vi "PicoErrorHandler2.vi"(7 "Mode":u16(ring) items=["Dialog On Error", "no dialog - CloseUnit and Stop", "no dialog - Continue", "no dialog - Stop"], 8 "error in (no error)":errorcluster={"status"=FALSE, "code"=0, "source"="0"}, 9 "PICO_STATUS in":T1={"status"=FALSE, "code"=0, "source"="NC"}, 10 "Default handle":i16=16384, 11 "handle In":i16=-1) -> (0 "error out":errorcluster)   [LabVIEW 2017]
doc: "This VI takes two inputs the \"error cluster\" and \"PICO_STATUS in\" if an error has occurred, displays a message box indicating the source of the error and the status code returned by the driver.\nAnd gives the option to close the handle to the API and stop the vi, \"continue\" or just \"stop\" the vi.\nThis can be over ridden using the \"Mode\" terminal as follows-\n0 = Dialog box On Error (Default)\n1 = CloseUnit and Stop\n2 = Continue \n3 = Stop\nIf \"PICO_STATUS in\" is not connected in the case with legacy code the \"error cluster\" value will be used.\nThe error cluster will passed unless it closes the API handle in which case the error cluster will be cleared.\nNote: The \"source\" terminal from the select cluster (\"error cluster\" or \"PICO_STATUS in\") is used to select which API close Unit function to call. If none match all are called."
panel:
  out "PICO_STATUS out":T1
  in  "Pico API list":string[](array[string])=["PLCM3", "UsbPt104", "ps2000a", "ps3000a", "ps4000a", "ps5000a", "ps6000a", "ps2000", "ps3000", "ps4000", "ps5000", "ps6000", "psospa"]
  out "CloseUnit Statuses":T2
  out "Pass or Unknown string":string
  out "Error String":string
  out "handle out":i16=16384
  in  "no error":errorcluster
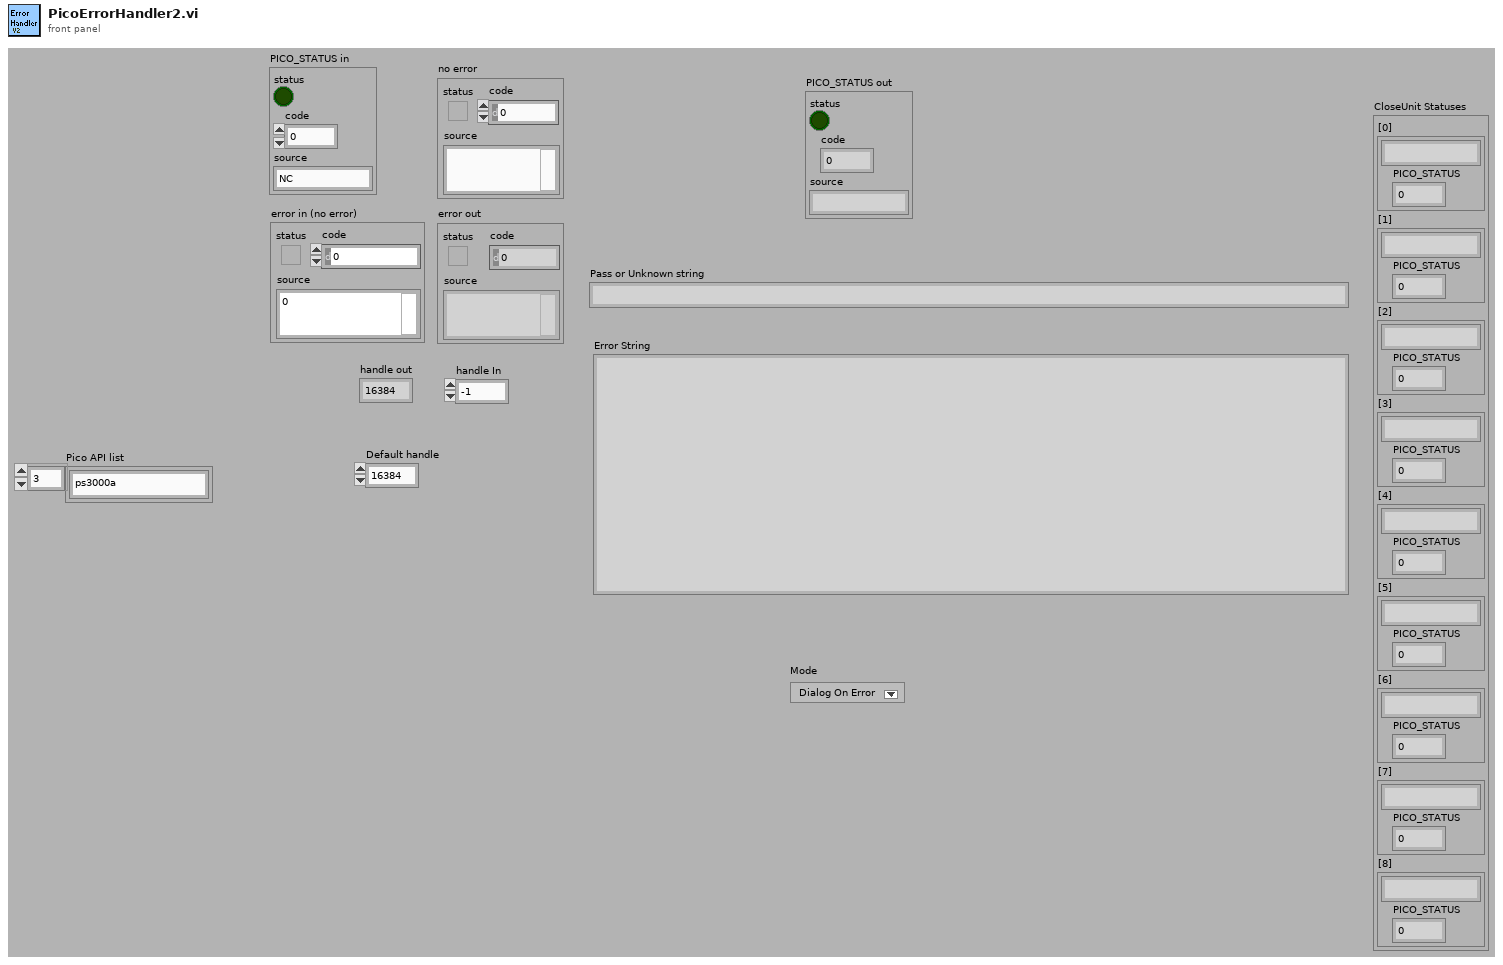
[diagram p1: front panel]
types:
  T1 = cluster{"status":bool, "code":u32, "source":string}
  T2 = cluster{"[0]":cluster{string, "PICO_STATUS":u32}, "[1]":cluster{string, "PICO_STATUS":u32}, "[2]":cluster{string, "PICO_STATUS":u32}, "[3]":cluster{string, "PICO_STATUS":u32}, "[4]":cluster{string, "PICO_STATUS":u32}, "[5]":cluster{string, "PICO_STATUS":u32}, "[6]":cluster{string, "PICO_STATUS":u32}, "[7]":cluster{string, "PICO_STATUS":u32}, "[8]":cluster{string, "PICO_STATUS":u32}}
  T3 = enum16{"Left Button", "Center Button", "Right Button", "Window Close"}
  T4 = cluster{"status":bool, "code":u32, "source":string}[]
  T5 = cluster{"[0]":cluster{"source":string, "PICO_STATUS":u32}, "[1]":cluster{"source":string, "PICO_STATUS":u32}, "[2]":cluster{"source":string, "PICO_STATUS":u32}, "[3]":cluster{"source":string, "PICO_STATUS":u32}, "[4]":cluster{"source":string, "PICO_STATUS":u32}, "[5]":cluster{"source":string, "PICO_STATUS":u32}, "[6]":cluster{"source":string, "PICO_STATUS":u32}, "[7]":cluster{"source":string, "PICO_STATUS":u32}, "[8]":cluster{"source":string, "PICO_STATUS":u32}}
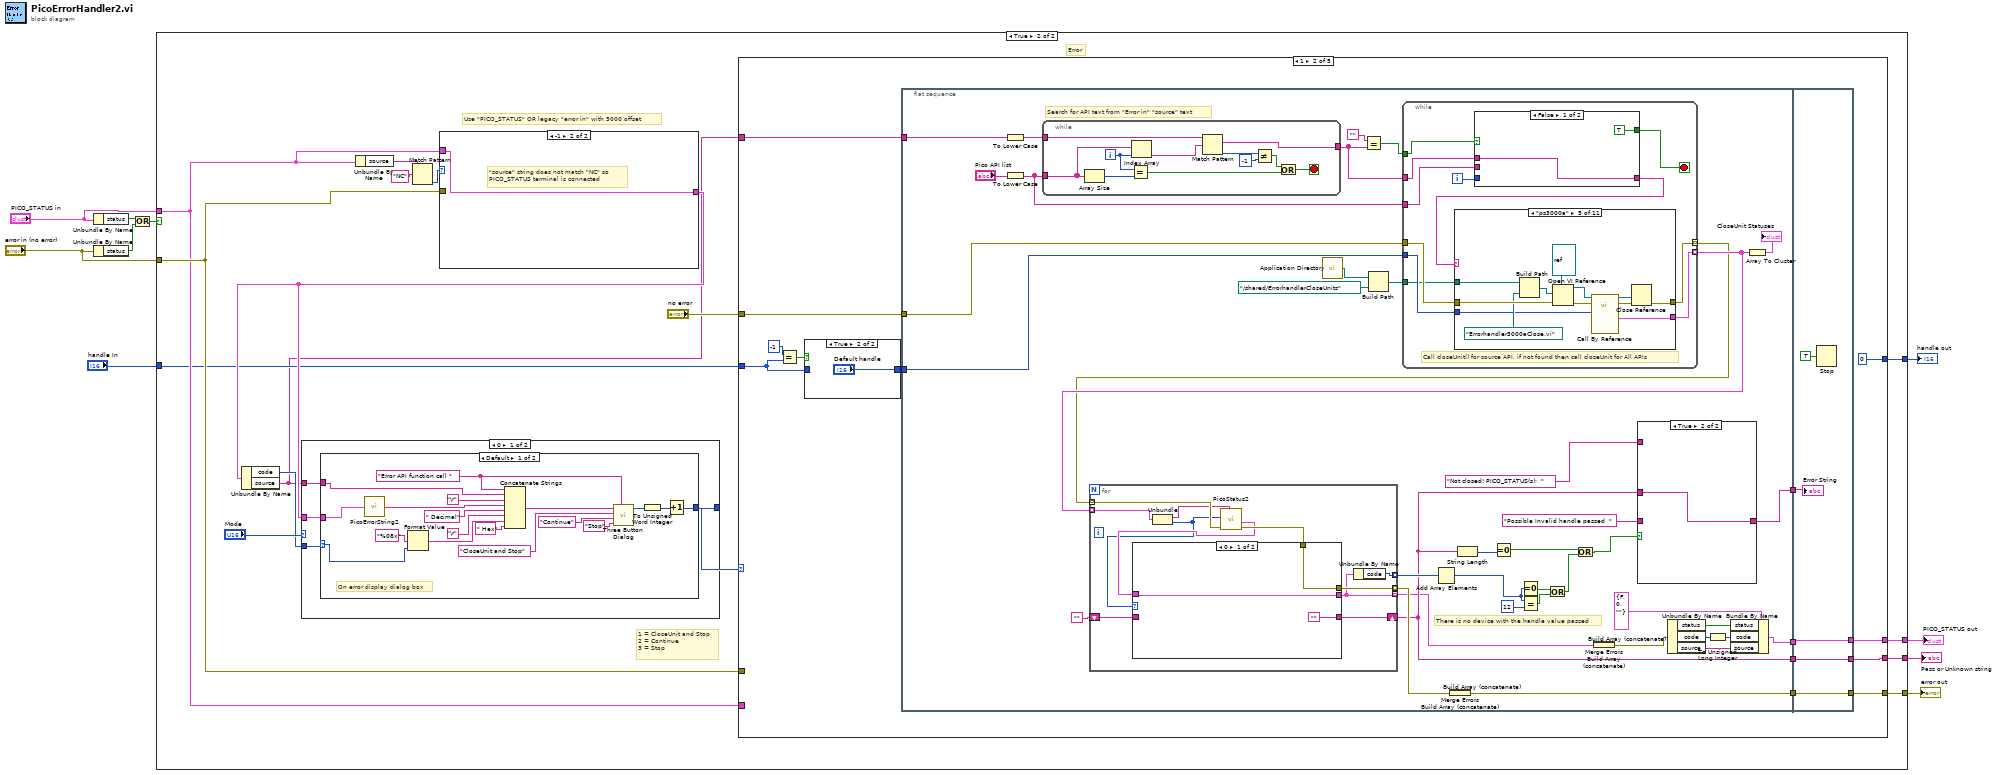
[diagram p0: block diagram]
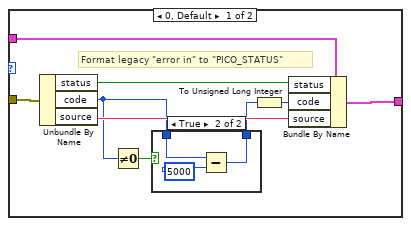
[diagram p3: hidden frame]
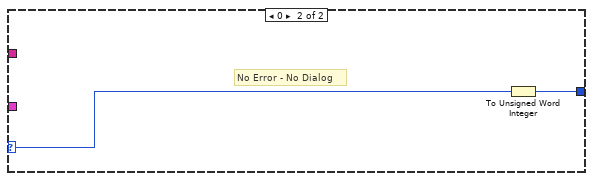
[diagram p5: hidden frame]
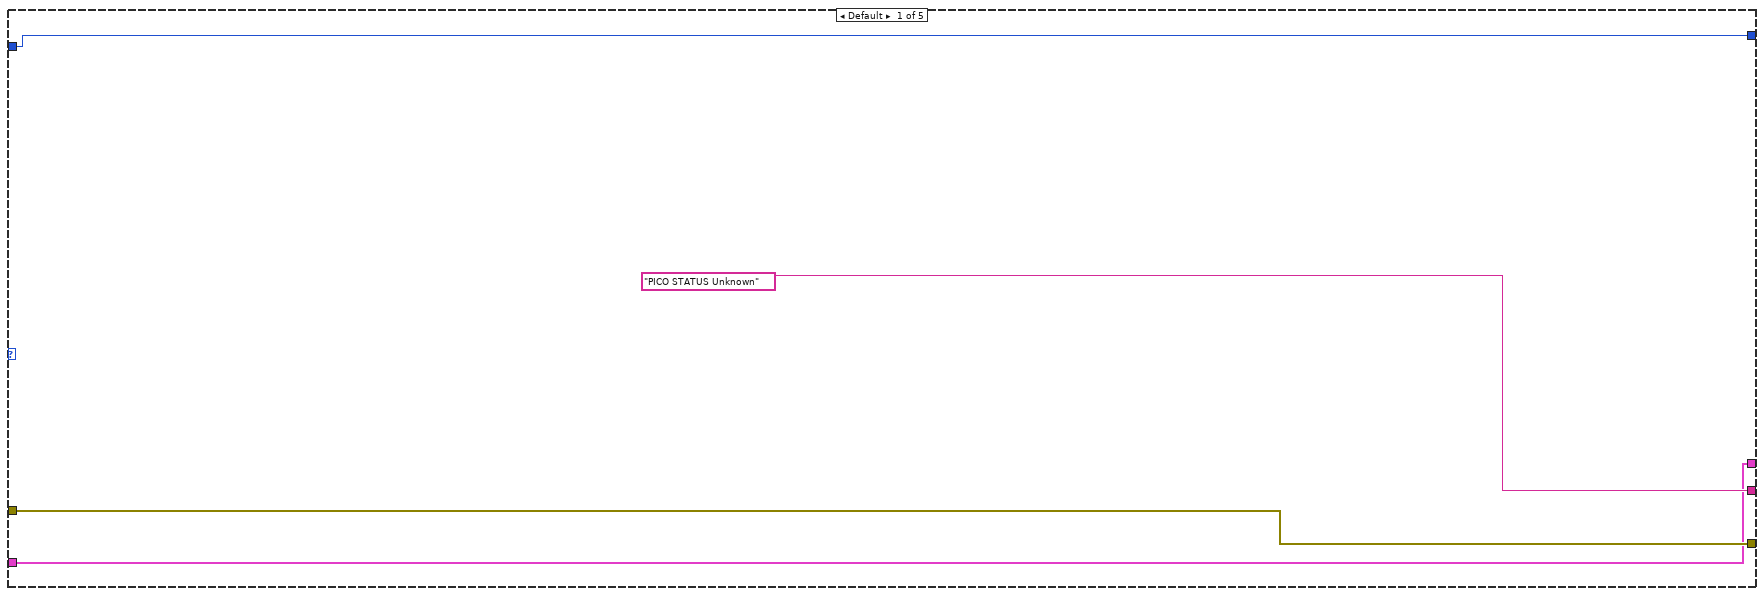
[diagram p7: hidden frame]
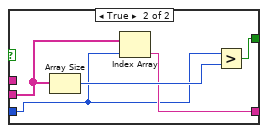
[diagram p9: hidden frame]
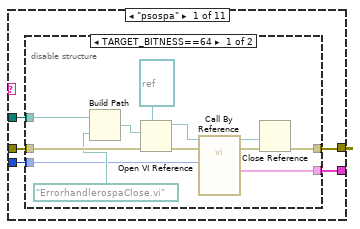
[diagram p10: hidden frame]
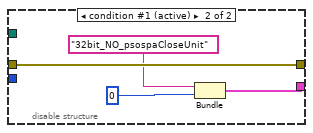
[diagram p11: hidden frame]
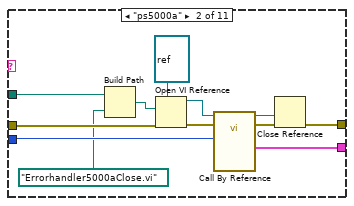
[diagram p12: hidden frame]
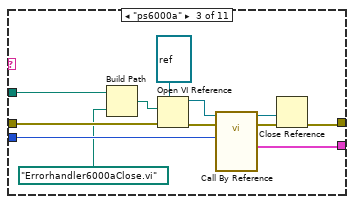
[diagram p13: hidden frame]
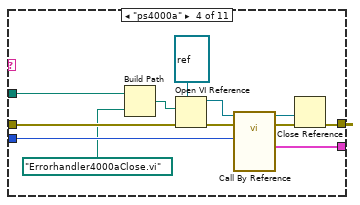
[diagram p14: hidden frame]
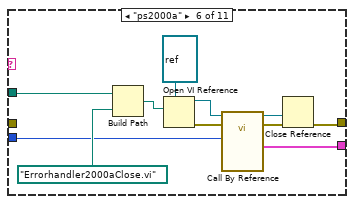
[diagram p15: hidden frame]
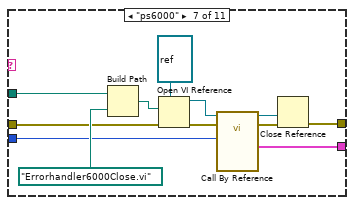
[diagram p16: hidden frame]
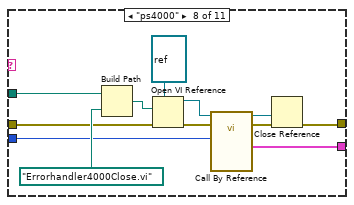
[diagram p17: hidden frame]
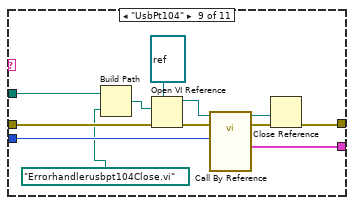
[diagram p18: hidden frame]
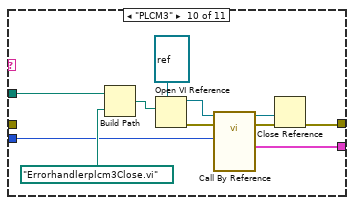
[diagram p19: hidden frame]
diagram:
  n1 = Unbundle By Name("PICO_STATUS in") -> ("status"=w2:bool)
  n2 = Unbundle By Name("error in (no error)") -> ("status"=w3:bool)
  n3 = Or(x=w2, y=w3) -> (x .or. y?=w1:bool)
  n4 = case shown="True" w1 {
    tunnel: "error in (no error)" -> [w13 w25]
    tunnel: "PICO_STATUS in" -> [w12 w20]
    tunnel: "handle In" -> [w11 w19]
    tunnel: [w12 w17] -> w9
    tunnel: [_ w16] -> w8
    tunnel: [w13 w15] -> w7
    tunnel: [w11 w14] -> w6
    frame False {
      # "No Error"
    }
    frame True {
      # "Error"
      # "Use \"PICO_STATUS\" OR legacy \"error in\" with 5000 offset"
      # "1 = CloseUnit and Stop\n2 = Continue \n3 = Stop"
      n5 = Unbundle By Name(w20) -> ("source"=w23:string)
      n6 = Match Pattern(string=w23, regular expression="NC") -> (offset past match=w21:i32)  [unwired: 1 in, 3 out]
      n7 = case shown="-1" w21 {
        tunnel: [w38 w43] -> w24
        tunnel: w25 -> [w35 _]
        tunnel: w20 -> [w32 w43]
        frame 0, Default {
          # "Format legacy \"error in\" to \"PICO_STATUS\""
          n8 = Unbundle By Name(w35) -> ("status"=w37:bool, "code"=w33:i32, "source"=w36:string)
          n9 = Not Equal To 0?(x=w33) -> (x != 0?=w34:bool)
          n10 = case shown="True" w34 {
            tunnel: w33 -> [w39 w41]
            tunnel: [w39 w40] -> w30
            frame False {
            }
            frame True {
              n11 = Subtract(x=w41, y=5000) -> (x-y=w40:i32)
            }
          }
          n12 = To Unsigned Long Integer(number=w30) -> (unsigned 32bit integer=w31:u32)
          n13 = Bundle By Name(cluster=w32, "status"=w37, "code"=w31, "source"=w36) -> (w38:T1)
        }
        frame -1 {
          # "\"source\" string does not match \"NC\" so\nPICO_STATUS terminal is connected"
        }
      }
      n14 = Unbundle By Name(w24) -> ("code"=w26:u32, "source"=w18:string)
      n15 = case shown="0" "Mode" {
        selector: "Mode" -> [_ w68]
        tunnel: w24 -> [w47 _]
        tunnel: w18 -> [w46 _]
        tunnel: [w45 w68] -> w28
        tunnel: w26 -> [w44 _]
        frame 0 {
          n16 = case shown="Default" w44 {
            selector: w44 -> [w48 w66]
            tunnel: w46 -> [w57 _]
            tunnel: [w60 w67] -> w45
            tunnel: w47 -> [w55 _]
            frame Default {
              w61 = "Error API function call "
              # "On error display dialog box"
              n17 = call "PicoErrorString2.vi"("PICO_STATUS in"=w55) -> ("String"=w54:string)  [unwired: 2 in, 2 out]
              n18 = Format Value(format string="%08x", value (0)=w48) -> (output string=w51:string)  [unwired: 1 in]
              n19 = Concatenate Strings(w61, w57, "\r", w54, " Decimal", "\r", w51, " Hex") -> (w62:string)
              n20 = call <vilib>:"Three Button Dialog.vi"("Window Title (\"\")"=w61, "Right Button Text (\"Cancel\")"="Stop" ("Right Button Text (\"Cancel\")"), "Center Button Text (\"No\")"="Continue" ("Center Button Text (\"No\")"), "Left Button Text (\"Yes\")"="CloseUnit and Stop" ("Left Button Text (\"Yes\")"), "message"=w62) -> ("Which Button?"=w58:T3)  [unwired: 6 in]
              n21 = To Unsigned Word Integer(number=w58) -> (unsigned 16bit integer=w59:u16)
              n22 = Increment(x=w59) -> (x+1=w60:u16)
            }
            frame 0 {
              # "No Error - No Dialog"
              n23 = To Unsigned Word Integer(number=w66) -> (unsigned 16bit integer=w67:u16)
            }
          }
        }
        frame 1, Default {
          # "No Dialog - Pass Mode"
        }
      }
      n24 = case shown="1" w28 {
        tunnel: ["PICO STATUS Unknown" w86 "Continue" ("Center Button Text (\"No\")") "Stop" ("Right Button Text (\"Cancel\")") "No Error Continue PICO_STATUS  is OK (0)" ("Center Button Text (\"No\")")] -> w16
        tunnel: [w71 w80 w324 w328 w333] -> w15
        tunnel: [w69 i16 0 ("handle In") w322 w326 w331] -> w14
        tunnel: w25 -> [w71 _ w324 w328 w333]
        tunnel: "no error" -> [_ w81 _ _ _]
        tunnel: [w70 w78 w323 w327 w332] -> w17
        tunnel: w20 -> [w70 _ w323 w327 w332]
        tunnel: w19 -> [w69 w75 w322 w326 w331]
        tunnel: w18 -> [_ w73 _ _ _]
        frame Default {
        }
        frame 1 {
          n25 = Equal?(x=i16 -1, y=w75) -> (x = y?=w77:bool)
          n26 = case shown="True" w77 {
            tunnel: w75 -> [w87 _]
            tunnel: [w87 "Default handle"] -> w74
            frame False {
            }
            frame True {
            }
          }
          n27 = flat-sequence {
            tunnel: w74 -> [w120]
            tunnel: [w113] -> w85
            tunnel: [w106] -> w84
            tunnel: [w129] -> w83
            tunnel: w81 -> [w103]
            tunnel: [w117] -> w79
            tunnel: w73 -> [w100]
            tunnel: [w320] -> w78
            tunnel: [w321] -> w86
            tunnel: w85 -> [w321]
            tunnel: w84 -> [w320]
            tunnel: w83 -> [w318]
            tunnel: [w317] -> w80
            tunnel: w79 -> [w317]
            frame #0 {
              # "Search for API text from \"Error in\" \"source\" text"
              # "There is no device with the handle value passed"
              n28 = To Lower Case(string=w100) -> (all lower case string=w101:string)
              n29 = To Lower Case(string="Pico API list") -> (all lower case string=w97:string[])
              n30 = while {
                tunnel: w101 -> [w133]
                tunnel: [w142] -> w96
                tunnel: w97 -> [w139]
                i -> [w137]
                stop <- w134 stop-if-true
                n31 = Array Size(array=w139) -> (size(s)=w138:i32)
                n32 = Equal?(x=w137, y=w138) -> (x = y?=w136:bool)
                n33 = Index Array(array=w139, index=w137) -> (element=w132:string)
                n34 = Match Pattern(string=w133, regular expression=w132) -> (match substring=w142:string, offset past match=w141:i32)  [unwired: 1 in, 2 out]
                n35 = Not Equal?(x=w141, y=-1) -> (x != y?=w135:bool)
                n36 = Or(x=w135, y=w136) -> (x .or. y?=w134:bool)
              }
              n37 = call <vilib>:"Application Directory.vi"() -> ("Application Directory"=w91:path)
              n38 = Equal?(x="", y=w96) -> (x = y?=w98:bool)
              n39 = Build Path(base path=w91, name or relative path=path "../shared/ErrorhandlerCloseUnits" ("vi path")) -> (appended path=w95:path)
              n40 = while {
                tunnel: w96 -> [w149]
                tunnel: w120 -> [w153]
                tunnel: [w144] -> w119 mode=indexing
                tunnel: w103 -> [w151]
                tunnel: [w152] -> w116 mode=indexing
                tunnel: w98 -> [w147]
                tunnel: w97 -> [w145]
                tunnel: w95 -> [w143]
                i -> [w146]
                stop <- w148 stop-if-true
                # "Call closeUnit() for source API, if not found then call closeUnit for All APIs"
                n41 = case shown="False" w147 {
                  tunnel: [w154 w158] -> w150
                  tunnel: w149 -> [w154 _]
                  tunnel: w146 -> [_ w157]
                  tunnel: [TRUE w160] -> w148
                  tunnel: w145 -> [_ w156]
                  frame False {
                  }
                  frame True {
                    n42 = Array Size(array=w156) -> (size(s)=w159:i32)
                    n43 = Index Array(array=w156, index=w157) -> (element=w158:string)
                    n44 = Greater?(x=w157, y=w159) -> (0:w160:bool)
                  }
                }
                n45 = case shown="\"ps3000a\"" w150 {
                  tunnel: w151 -> [w165 w183 w198 w217 w221 _ w244 w254 w266 _ w288]
                  tunnel: w153 -> [w164 w184 w197 w208 w218 w230 w243 w255 w267 w277 _]
                  tunnel: [w163 w186 w195 w216 w223 w232 w241 w257 w269 w279 w288] -> w152
                  tunnel: [w162 w185 w196 w207 w219 w231 w242 w253 w268 w278 _] -> w144
                  tunnel: w143 -> [w161 w187 w199 w214 w222 w234 w246 w258 w270 w281 _]
                  frame "psospa" {
                    n46 = disable-structure shown="TARGET_BITNESS==64" {
                      disable-tunnel: [w167 w179] -> w162
                      disable-tunnel: [w166 w181] -> w163
                      disable-tunnel: w165 -> [w170 w181]
                      disable-tunnel: w164 -> [w168 _]
                      disable-tunnel: w161 -> [w171 _]
                      frame condition #0 {
                        n47 = Build Path(base path=w171, name or relative path=path "ErrorhandlerospaClose.vi" ("vi path")) -> (appended path=w176:path)
                        n48 = Open VI Reference(type specifier VI Refnum (for type only)=refnum<vi> refnum, vi path=w176, error in (no error)=w170) -> (vi reference=w175:refnum<vi>, error out=w174:errorcluster)  [unwired: 3 in]
                        n49 = call-by-ref "?"(reference=w175, error in=w174, "handle in"=w168) -> (reference out=w172:refnum<vi>, error out=w173:errorcluster, "output cluster"=w167:cluster{"source":string, "PICO_STATUS":u32})  [unwired: 8 in, 2 out]
                        n50 = Close Reference(reference=w172, error in (no error)=w173) -> (error out=w166:errorcluster)
                      }
                      frame condition #1 (active) {
                        n51 = Bundle("source"="32bit_NO_psospaCloseUnit", "handle out"=i16 0) -> (w179:cluster{"source":string, "handle out":i16})  [unwired: 1 in]
                      }
                    }
                  }
                  frame "ps5000a" {
                    n52 = Build Path(base path=w187, name or relative path=path "Errorhandler5000aClose.vi" ("vi path")) -> (appended path=w192:path)
                    n53 = Open VI Reference(type specifier VI Refnum (for type only)=refnum<vi> refnum, vi path=w192, error in (no error)=w183) -> (vi reference=w191:refnum<vi>, error out=w190:errorcluster)  [unwired: 3 in]
                    n54 = call-by-ref "?"(reference=w191, error in=w190, "handle in"=w184) -> (reference out=w188:refnum<vi>, error out=w189:errorcluster, "output cluster"=w185:cluster{"source":string, "PICO_STATUS":u32})  [unwired: 8 in, 2 out]
                    n55 = Close Reference(reference=w188, error in (no error)=w189) -> (error out=w186:errorcluster)
                  }
                  frame "ps6000a" {
                    n56 = Build Path(base path=w199, name or relative path=path "Errorhandler6000aClose.vi" ("vi path")) -> (appended path=w204:path)
                    n57 = Open VI Reference(type specifier VI Refnum (for type only)=refnum<vi> refnum, vi path=w204, error in (no error)=w198) -> (vi reference=w203:refnum<vi>, error out=w202:errorcluster)  [unwired: 3 in]
                    n58 = call-by-ref "?"(reference=w203, error in=w202, "handle in"=w197) -> (reference out=w200:refnum<vi>, error out=w201:errorcluster, "output cluster"=w196:cluster{"source":string, "PICO_STATUS":u32})  [unwired: 8 in, 2 out]
                    n59 = Close Reference(reference=w200, error in (no error)=w201) -> (error out=w195:errorcluster)
                  }
                  frame "ps4000a" {
                    n60 = Build Path(base path=w214, name or relative path=path "Errorhandler4000aClose.vi" ("vi path")) -> (appended path=w213:path)
                    n61 = Open VI Reference(type specifier VI Refnum (for type only)=refnum<vi> refnum, vi path=w213, error in (no error)=w217) -> (vi reference=w212:refnum<vi>, error out=w211:errorcluster)  [unwired: 3 in]
                    n62 = call-by-ref "?"(reference=w212, error in=w211, "handle in"=w208) -> (reference out=w209:refnum<vi>, error out=w210:errorcluster, "output cluster"=w207:cluster{"source":string, "PICO_STATUS":u32})  [unwired: 8 in, 2 out]
                    n63 = Close Reference(reference=w209, error in (no error)=w210) -> (error out=w216:errorcluster)
                  }
                  frame "ps3000a" {
                    n64 = Build Path(base path=w222, name or relative path=path "Errorhandler3000aClose.vi" ("vi path")) -> (appended path=w228:path)
                    n65 = Open VI Reference(type specifier VI Refnum (for type only)=refnum<vi> refnum, vi path=w228, error in (no error)=w221) -> (vi reference=w227:refnum<vi>, error out=w226:errorcluster)  [unwired: 3 in]
                    n66 = call-by-ref "?"(reference=w227, error in=w226, "handle in"=w218) -> (reference out=w224:refnum<vi>, error out=w225:errorcluster, "output cluster"=w219:cluster{"source":string, "PICO_STATUS":u32})  [unwired: 8 in, 2 out]
                    n67 = Close Reference(reference=w224, error in (no error)=w225) -> (error out=w223:errorcluster)
                  }
                  frame "ps2000a" {
                    n68 = Build Path(base path=w234, name or relative path=path "Errorhandler2000aClose.vi" ("vi path")) -> (appended path=w239:path)
                    n69 = Open VI Reference(type specifier VI Refnum (for type only)=refnum<vi> refnum, vi path=w239) -> (vi reference=w238:refnum<vi>, error out=w237:errorcluster)  [unwired: 4 in]
                    n70 = call-by-ref "?"(reference=w238, error in=w237, "handle in"=w230) -> (reference out=w235:refnum<vi>, error out=w236:errorcluster, "output cluster"=w231:cluster{"source":string, "PICO_STATUS":u32})  [unwired: 8 in, 2 out]
                    n71 = Close Reference(reference=w235, error in (no error)=w236) -> (error out=w232:errorcluster)
                  }
                  frame "ps6000" {
                    n72 = Build Path(base path=w246, name or relative path=path "Errorhandler6000Close.vi" ("vi path")) -> (appended path=w251:path)
                    n73 = Open VI Reference(type specifier VI Refnum (for type only)=refnum<vi> refnum, vi path=w251, error in (no error)=w244) -> (vi reference=w250:refnum<vi>, error out=w249:errorcluster)  [unwired: 3 in]
                    n74 = call-by-ref "?"(reference=w250, error in=w249, "handle in"=w243) -> (reference out=w247:refnum<vi>, error out=w248:errorcluster, "output cluster"=w242:cluster{"source":string, "PICO_STATUS":u32})  [unwired: 8 in, 2 out]
                    n75 = Close Reference(reference=w247, error in (no error)=w248) -> (error out=w241:errorcluster)
                  }
                  frame "ps4000" {
                    n76 = Build Path(base path=w258, name or relative path=path "Errorhandler4000Close.vi" ("vi path")) -> (appended path=w259:path)
                    n77 = Open VI Reference(type specifier VI Refnum (for type only)=refnum<vi> refnum, vi path=w259, error in (no error)=w254) -> (vi reference=w263:refnum<vi>, error out=w262:errorcluster)  [unwired: 3 in]
                    n78 = call-by-ref "?"(reference=w263, error in=w262, "handle in"=w255) -> (reference out=w260:refnum<vi>, error out=w261:errorcluster, "output cluster"=w253:cluster{"source":string, "PICO_STATUS":u32})  [unwired: 8 in, 2 out]
                    n79 = Close Reference(reference=w260, error in (no error)=w261) -> (error out=w257:errorcluster)
                  }
                  frame "UsbPt104" {
                    n80 = Build Path(base path=w270, name or relative path=path "Errorhandlerusbpt104Close.vi" ("vi path")) -> (appended path=w275:path)
                    n81 = Open VI Reference(type specifier VI Refnum (for type only)=refnum<vi> refnum, vi path=w275, error in (no error)=w266) -> (vi reference=w274:refnum<vi>, error out=w273:errorcluster)  [unwired: 3 in]
                    n82 = call-by-ref "?"(reference=w274, error in=w273, "handle in"=w267) -> (reference out=w271:refnum<vi>, error out=w272:errorcluster, "output cluster"=w268:cluster{"source":string, "PICO_STATUS":u32})  [unwired: 8 in, 2 out]
                    n83 = Close Reference(reference=w271, error in (no error)=w272) -> (error out=w269:errorcluster)
                  }
                  frame "PLCM3" {
                    n84 = Build Path(base path=w281, name or relative path=path "Errorhandlerplcm3Close.vi" ("vi path")) -> (appended path=w286:path)
                    n85 = Open VI Reference(type specifier VI Refnum (for type only)=refnum<vi> refnum, vi path=w286) -> (vi reference=w285:refnum<vi>, error out=w284:errorcluster)  [unwired: 4 in]
                    n86 = call-by-ref "?"(reference=w285, error in=w284, "handle in"=w277) -> (reference out=w282:refnum<vi>, error out=w283:errorcluster, "output cluster"=w278:cluster{"source":string, "PICO_STATUS":u32})  [unwired: 8 in, 2 out]
                    n87 = Close Reference(reference=w282, error in (no error)=w283) -> (error out=w279:errorcluster)
                  }
                  frame "False", Default {
                  }
                }
              }
              n88 = for {
                shift-right: [w305] -> w113
                shift-left: "" -> [w306]
                tunnel: w119 -> [w303] mode=indexing
                tunnel: w116 -> [w298] mode=indexing
                tunnel: [w302] -> w105 mode=indexing
                tunnel: [w304] -> w118 mode=indexing
                tunnel: [w301] -> w115 mode=indexing
                n89 = Unbundle(w303) -> ("source"=w297:string, "PICO_STATUS"=w296:u32)
                n90 = call "PicoStatus2.vi"("PICO source"=w297, "Error in"=w298, "PICO STATUS"=w296) -> ("error out"=w300:errorcluster, "PICO_STATUS out"=w299:T1)  [unwired: 5 in]
                n91 = case shown="0" w296 {
                  tunnel: ["" w316] -> w305
                  tunnel: w306 -> [_ w315]
                  tunnel: w299 -> [w307 w311]
                  tunnel: [w307 w311] -> w302
                  tunnel: [w308 w310] -> w304
                  tunnel: w300 -> [w308 w310]
                  frame 0 {
                  }
                  frame Default {
                    n92 = call "PicoErrorString2.vi"("PICO_STATUS in"=w311) -> ("String"=w312:string)  [unwired: 2 in, 2 out]
                    n93 = call <vilib>:"Space Constant.vi"() -> ("String"=w314:string)
                    n94 = Concatenate Strings(w315, w314, w312, "\r") -> (w316:string)
                  }
                }
                n95 = Unbundle By Name(w302) -> ("code"=w301:u32)
              }
              n96 = Add Array Elements(numeric array=w115) -> (sum=w114:u32)
              n97 = Build Array (concatenate)(w118) -> (w92:errorcluster[])
              n98 = Build Array (concatenate)(w92) -> (w89:errorcluster[])
              n99 = Merge Errors(w89) -> (w117:errorcluster)
              n100 = String Length(string=w113) -> (length=w130:i32)
              n101 = Equal To 0?(x=w130) -> (x = 0?=w122:bool)
              n102 = Equal To 0?(x=w114) -> (x = 0?=w126:bool)
              n103 = Equal?(x=w114, y=u32 12) -> (x = y?=w125:bool)
              n104 = Or(x=w126, y=w125) -> (x .or. y?=w123:bool)
              n105 = Or(x=w122, y=w123) -> (x .or. y?=w121:bool)
              n106 = Build Array (concatenate)(w105) -> (w93:T4)
              n107 = Build Array (concatenate)(w93) -> (w90:T4)
              n108 = Merge Errors(w90) -> (w107:errorcluster)
              n109 = case shown="True" w121 {
                tunnel: [w293 w295] -> w129
                tunnel: w113 -> [w291 w295]
                tunnel: "Possible Invalid handle passed  " ("Left Button Text (\"Yes\")") -> [w294 _]
                tunnel: "Not closed! PICO_STATUS(s);  " ("Left Button Text (\"Yes\")") -> [w289 _]
                frame False {
                  # "Error"
                  n110 = Concatenate Strings(w289, "\r", w291) -> (w290:string)
                  n111 = Concatenate Strings(w290, w294) -> (w293:string)
                  n112 = One Button Dialog(message=w293) -> ()  [unwired: 1 in, 1 out]
                }
                frame True {
                }
              }
              n113 = Unbundle By Name(w107) -> ("status"=w108:bool, "code"=w111:i32, "source"=w109:string)
              n114 = To Unsigned Long Integer(number=w111) -> (unsigned 32bit integer=w110:u32)
              n115 = Bundle By Name(cluster=T1 {"status"=FALSE, "code"=0, "source"=""} ("PICO_STATUS in"), "status"=w108, "code"=w110, "source"=w109) -> (w106:T1)
              n116 = Array To Cluster(array=w119) -> (cluster=→"CloseUnit Statuses":T5)
            }
            frame #1 {
              n117 = Stop(stop? (T)=TRUE) -> ()
              "Error String" <- w318
            }
          }
        }
        frame 2 {
        }
        frame 3 {
          n118 = Stop(stop? (T)=TRUE) -> ()
        }
        frame 0 {
        }
      }
    }
  }
  "error out" <- w7
  "Pass or Unknown string" <- w8
  "PICO_STATUS out" <- w9
  "handle out" <- w6
